vi "CRYGet String Reference.vi"(10 "Label Name":string, 11 "VI Refnum":refnum<vi>) -> (1 "Find?":bool, 2 "String Ref Out":refnum<vi>, 3 "VI Refnum Out":refnum<vi>)   [LabVIEW 2013]
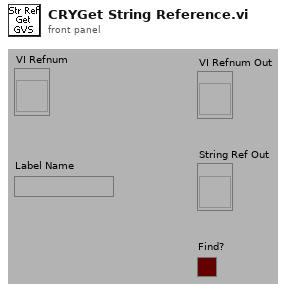
[diagram p1: front panel]
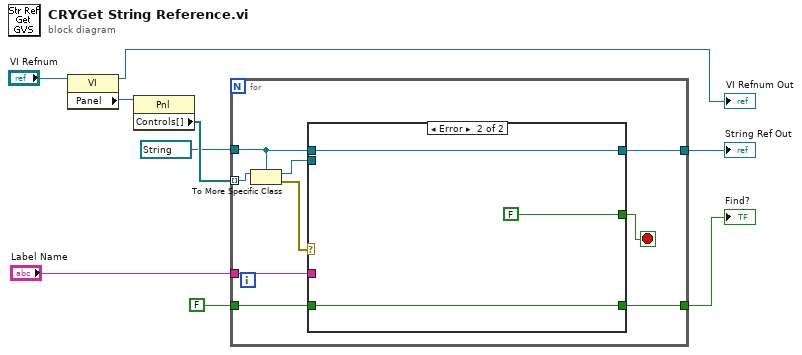
[diagram p0: block diagram]
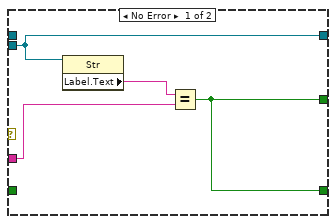
[diagram p2: hidden frame]
diagram:
  n1 = property class="VI"(reference="VI Refnum") -> (reference out=→"VI Refnum Out":refnum<vi>, "Panel"=w2:refnum<vi>)  [unwired: 1 in, 1 out]
  n2 = property class="Pnl"(reference=w2) -> ("Controls[]"=w8:refnum<vi>[])  [unwired: 1 in, 2 out]
  n3 = for {
    tunnel: w8 -> [w18] mode=indexing
    tunnel: [w14] -> w5
    tunnel: "Label Name" -> [w13]
    tunnel: refnum<vi> refnum ("ControlType") -> [w12]
    tunnel: FALSE ("Boolean") -> [w11]
    tunnel: [w10] -> w3
    stop <- w15 stop-if-true
    n4 = To More Specific Class(target class=w12, reference=w18) -> (specific class reference=w16:refnum<vi>, error out=w17:errorcluster)  [unwired: 1 in]
    n5 = case shown="Error" w17 {
      tunnel: w16 -> [w20 _]
      tunnel: [w19 FALSE] -> w15
      tunnel: [w20 w24] -> w14
      tunnel: w13 -> [w21 _]
      tunnel: w12 -> [_ w24]
      tunnel: [w19 w23] -> w10
      tunnel: w11 -> [_ w23]
      frame No Error {
        n6 = property class="Str"(reference=w20) -> ("Label.Text"=w22:string)  [unwired: 1 in, 2 out]
        n7 = Equal?(x=w22, y=w21) -> (x = y?=w19:bool)
      }
      frame Error {
      }
    }
  }
  "Find?" <- w3
  "String Ref Out" <- w5
